vi "Conversor de sinal.vi"(11 "Signal Type":string) -> (3 "Signal Type Out":T1(ring))   [LabVIEW 2020]
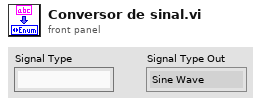
[diagram p1: front panel]
types:
  T1 = enum16{"Sine Wave", "Triangle Wave", "Square Wave", "Sawtooth Wave"}
  T2 = enum16{"Sine Wave", "Triangle Wave", "Square Wave", "Sawtooth Wave"}[]
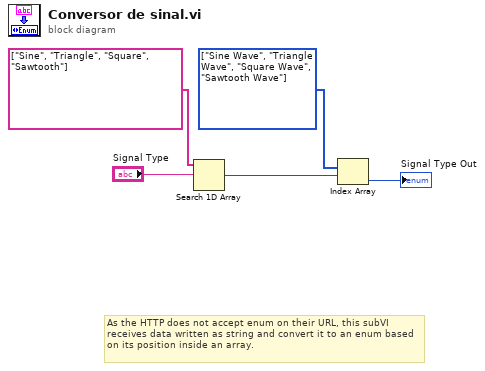
[diagram p0: block diagram]
diagram:
  w4 = T2 [enum."Sine Wave", enum."Triangle Wave", enum."Square Wave", enum."Sawtooth Wave"] items=["Sine Wave", "Triangle Wave", "Square Wave", "Sawtooth Wave"] ("signal type")
  # "As the HTTP does not accept enum on their URL, this subVI receives data written as string and convert it to an enum based on its position inside an array."
  n1 = Search 1D Array(1D array=string[] ["Sine", "Triangle", "Square", "Sawtooth"], element="Signal Type") -> (index of element=w3:i32)  [unwired: 1 in]
  n2 = Index Array(array=w4, index=w3) -> (element=→"Signal Type Out":T1)
